vi "MutationParentLevelsAdded.vi"(8 "error in (no error)":errorcluster, 10 "Parent Levels Added":u16, 11 "Object stack in (child, parent)":T1[](array[typedef])) -> (0 "error out":errorcluster, 2 "ClassOps":T2[](array[typedef]), 3 "Object stack out (child, parent)":T1[](array[typedef]))   [LabVIEW 2020, in "BlueSerialization.lvlib" / "BlueSerializer.lvclass"]
uses:
  BlueSerializer.lvclass
  Support/SetSerializableDataClusterIterable.ctl
  BlueSerializable/BlueSerializable.lvclass
  Support/SetSerializableDataClusterLayer.ctl
  BlueSerializableVersion.ctl
  Support/SetSerializableDataObject.ctl
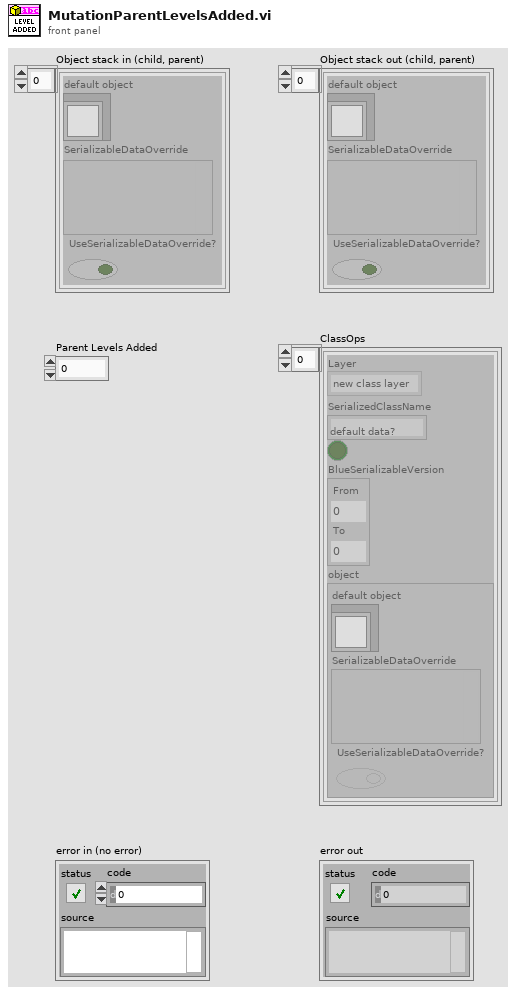
[diagram p1: front panel]
types:
  T1 = typedef "BlueSerialization.lvlib/BlueSerializer.lvclass/SetSerializableDataObject.ctl" = cluster{"default object":refnum<class "BlueSerializable.lvclass">, "SerializableDataOverride":variant, "UseSerializableDataOverride?":bool}
  T2 = typedef "BlueSerialization.lvlib/BlueSerializer.lvclass/SetSerializableDataClusterIterable.ctl" = cluster{"Layer":T3, "SerializedClassName":string, "default data?":bool, "BlueSerializableVersion":T4, "object":T1}
  T3 = typedef "BlueSerialization.lvlib/BlueSerializer.lvclass/SetSerializableDataClusterLayer.ctl" = enum16{"new class layer", "dropped class layer", "agreed class layer"}
  T4 = typedef "BlueSerialization.lvlib/BlueSerializer.lvclass/BlueSerializableVersion.ctl" = cluster{"From":u16, "To":u16}
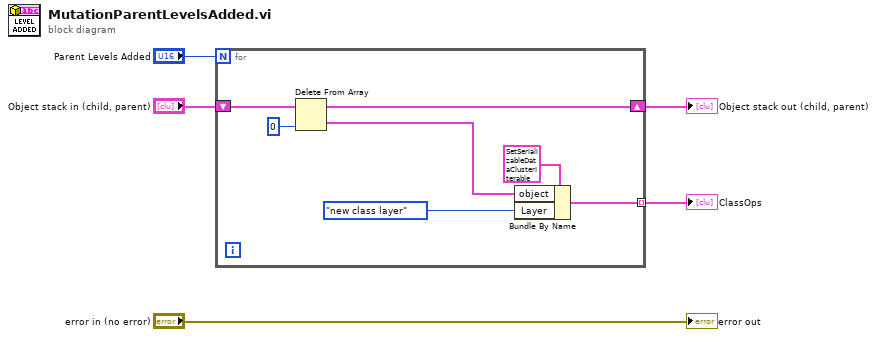
[diagram p0: block diagram]
diagram:
  n1 = for {
    N: "Parent Levels Added" -> [_]
    shift-right: [w10] -> w1
    shift-left: "Object stack in (child, parent)" -> [w11]
    tunnel: [w8] -> w3 mode=indexing
    n2 = Delete From Array(array=w11, index=0) -> (deleted portion=w6:T1, array with subset deleted=w10:T1[])  [unwired: 1 in]
    n3 = Bundle By Name(cluster=T2 {"Layer"=enum."new class layer", "SerializedClassName"="", "default data?"=FALSE, "BlueSerializableVersion"={"From"=0, "To"=0}, "object"={"default object"=refnum, "SerializableDataOverride"=variant(cluster{"SerializableData":variant, "Use?":bool} {"SerializableData"=variant, "Use?"=FALSE}), "UseSerializableDataOverride?"=FALSE}} ("Cluster 2"), "object"=w6, "Layer"=SetSerializableDataClusterLayer."new class layer") -> (w8:T2)
  }
  "ClassOps" <- w3
  "Object stack out (child, parent)" <- w1
  "error out" <- "error in (no error)"
